vi "Product.vi"(9 "Size":T1, 10 "Color":T2, 11 "Name":string) -> (3 "Product":refnum<class "Product.lvclass">)   [LabVIEW 2018, in "Product.lvclass"]
uses:
  Product.lvclass
  Color.ctl
  Size.ctl
  Product.lvclass/Product.ctl
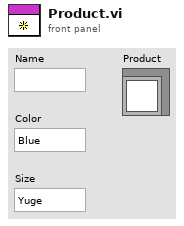
[diagram p1: front panel]
types:
  T1 = typedef "Product.lvclass/Size.ctl" = enum16{"Yuge", "Big", "Medium", "Small"}
  T2 = typedef "Product.lvclass/Color.ctl" = enum16{"Blue", "Green", "Red"}
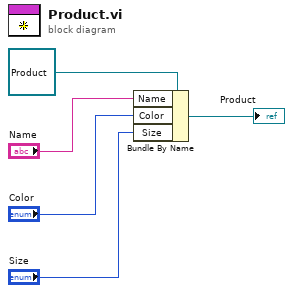
[diagram p0: block diagram]
diagram:
  n1 = Bundle By Name(cluster=refnum<class "Product.lvclass"> refnum ("Product in"), "Name"="Name", "Color"="Color", "Size"="Size") -> (→"Product":refnum<class "Product.lvclass">)
